vi "DisplayArm.vi"(4 "Init?":bool, 6 "ClosePt":dbl[](array[numeric]), 7 "Field Force":dbl[](array[numeric]), 8 "AnkleTraj":dbl[][](array[numeric]), 9 "CablePos":cluster{"PointInGCS":dbl[][]}[](array[cluster]), 10 "Joint Coord in GCS":dbl[][](array[numeric]), 11 "3D graph in":refnum<k7>) -> (3 "3D graph out":refnum<k7>)   [LabVIEW 2014]
uses:
  <vilib>/Platform/NI_3dgraph.lvlib
  <vilib>/ptbypt/NI_PtbyPt.lvlib
panel:
  in  "sample length":i32=100
  out "LastPlotNum":i32=1
  out "error out":errorcluster
  in  "error in (no error)":errorcluster
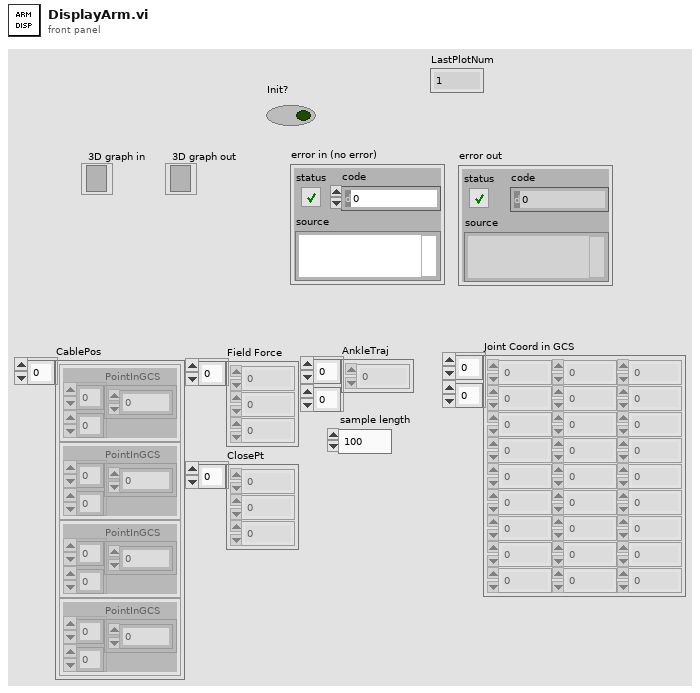
[diagram p1: front panel]
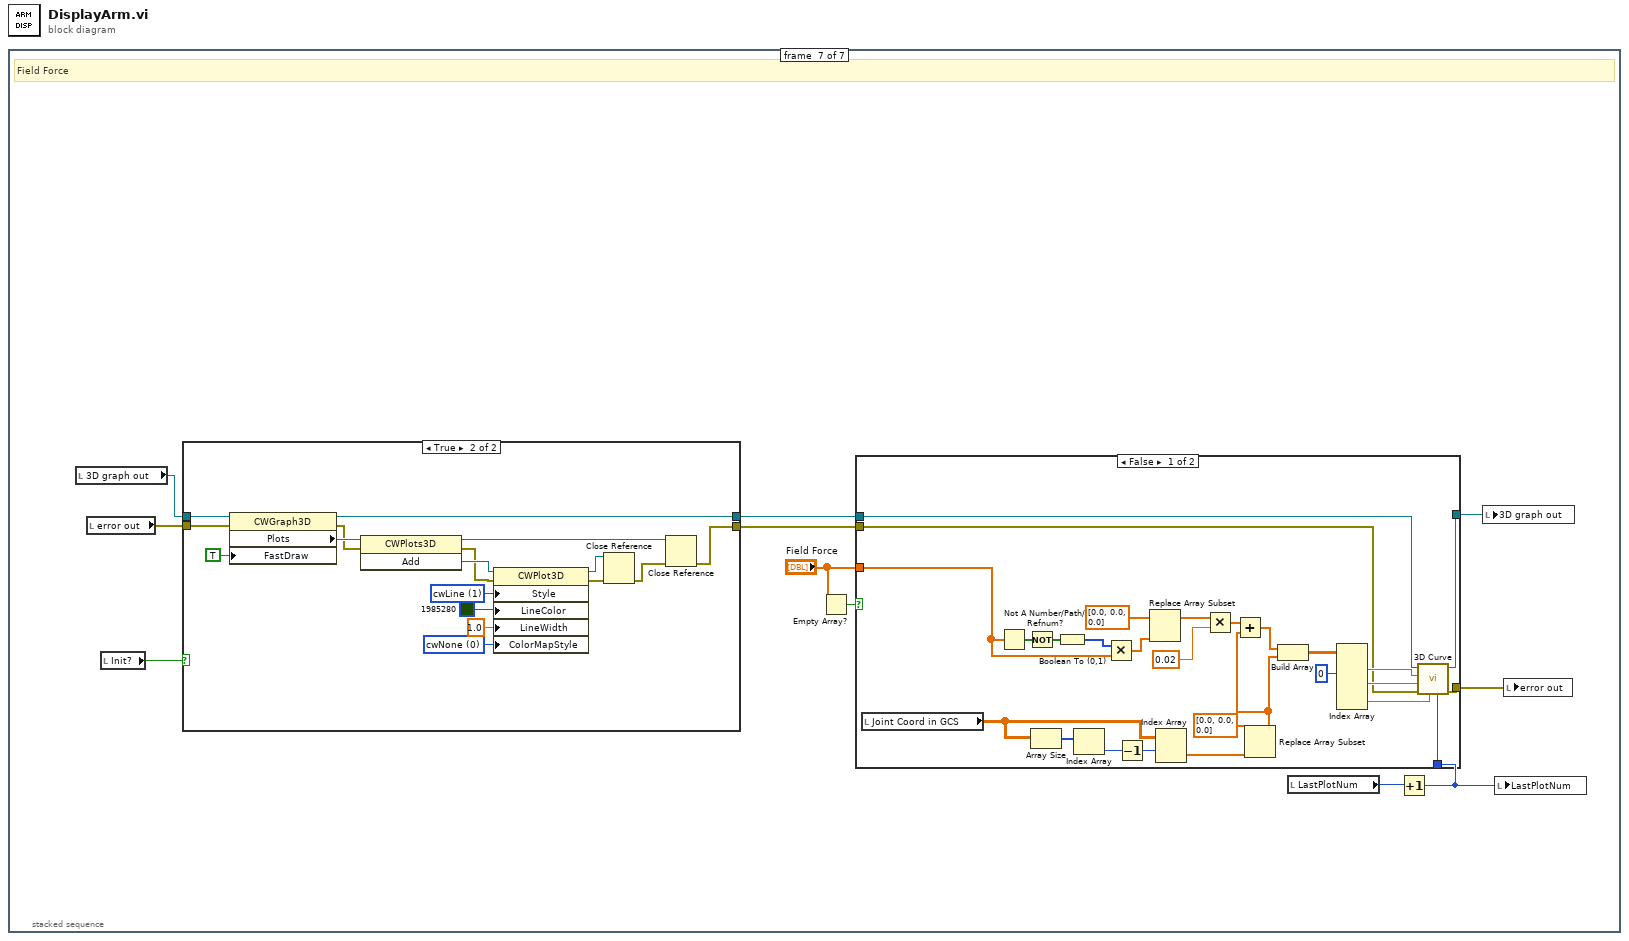
[diagram p0: block diagram]
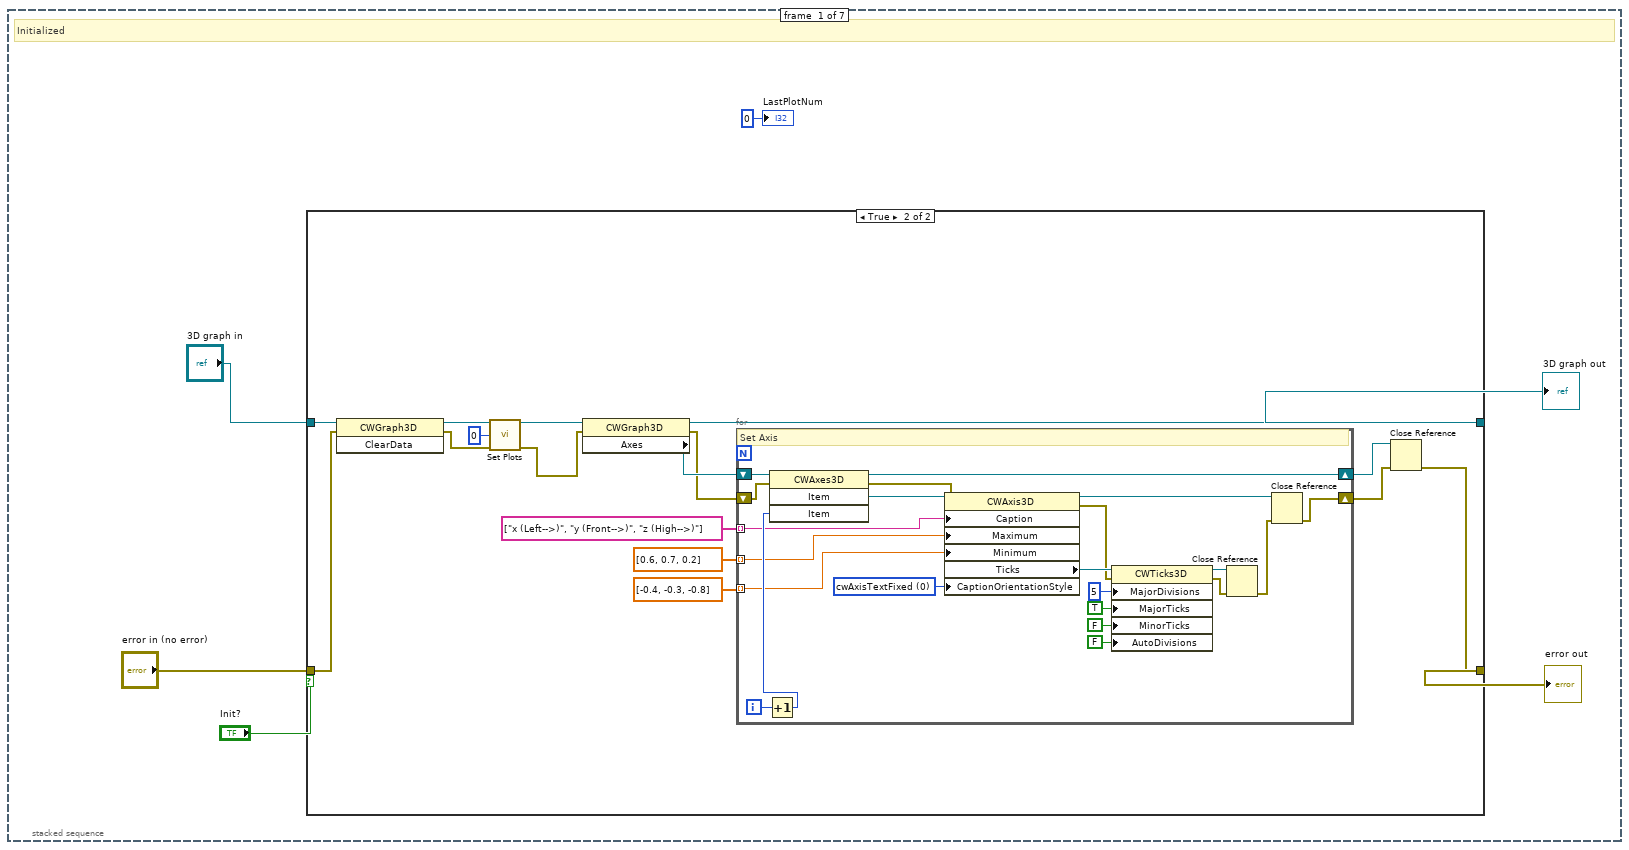
[diagram p2: hidden frame]
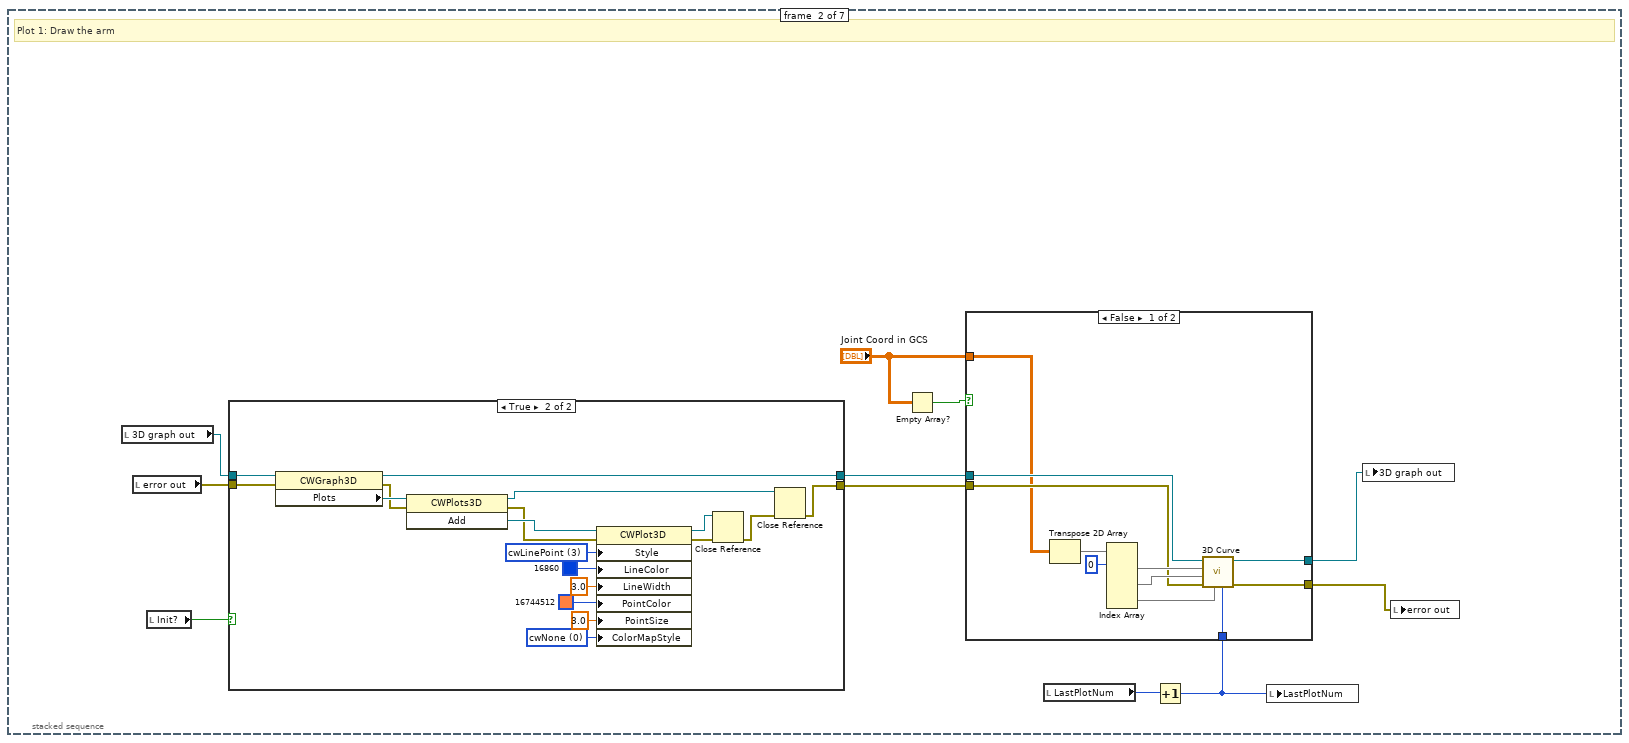
[diagram p4: hidden frame]
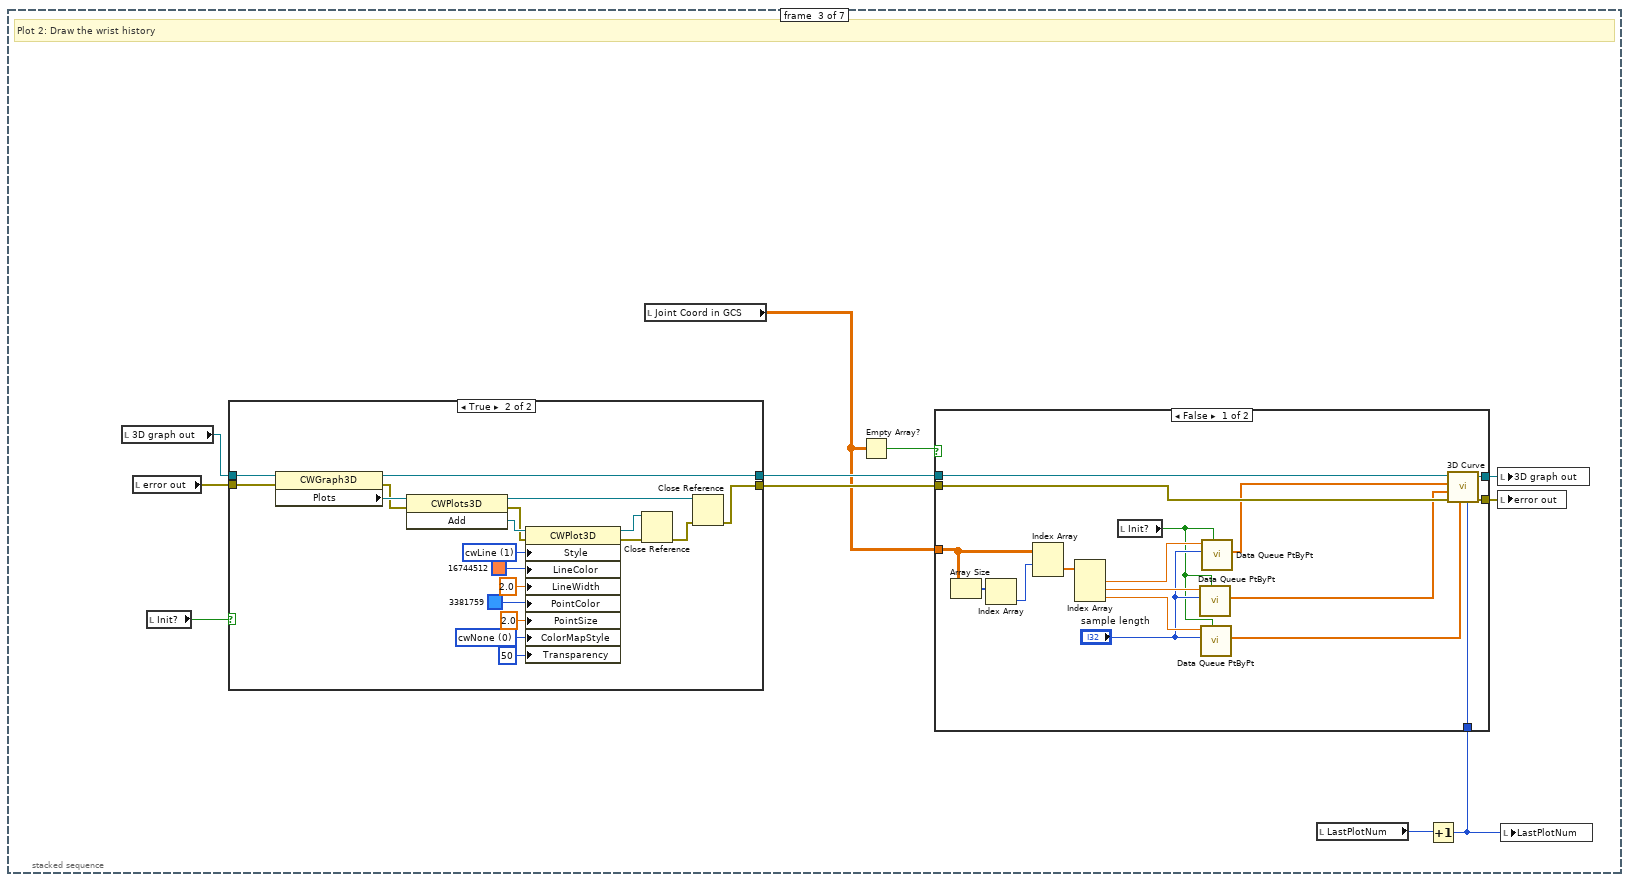
[diagram p7: hidden frame]
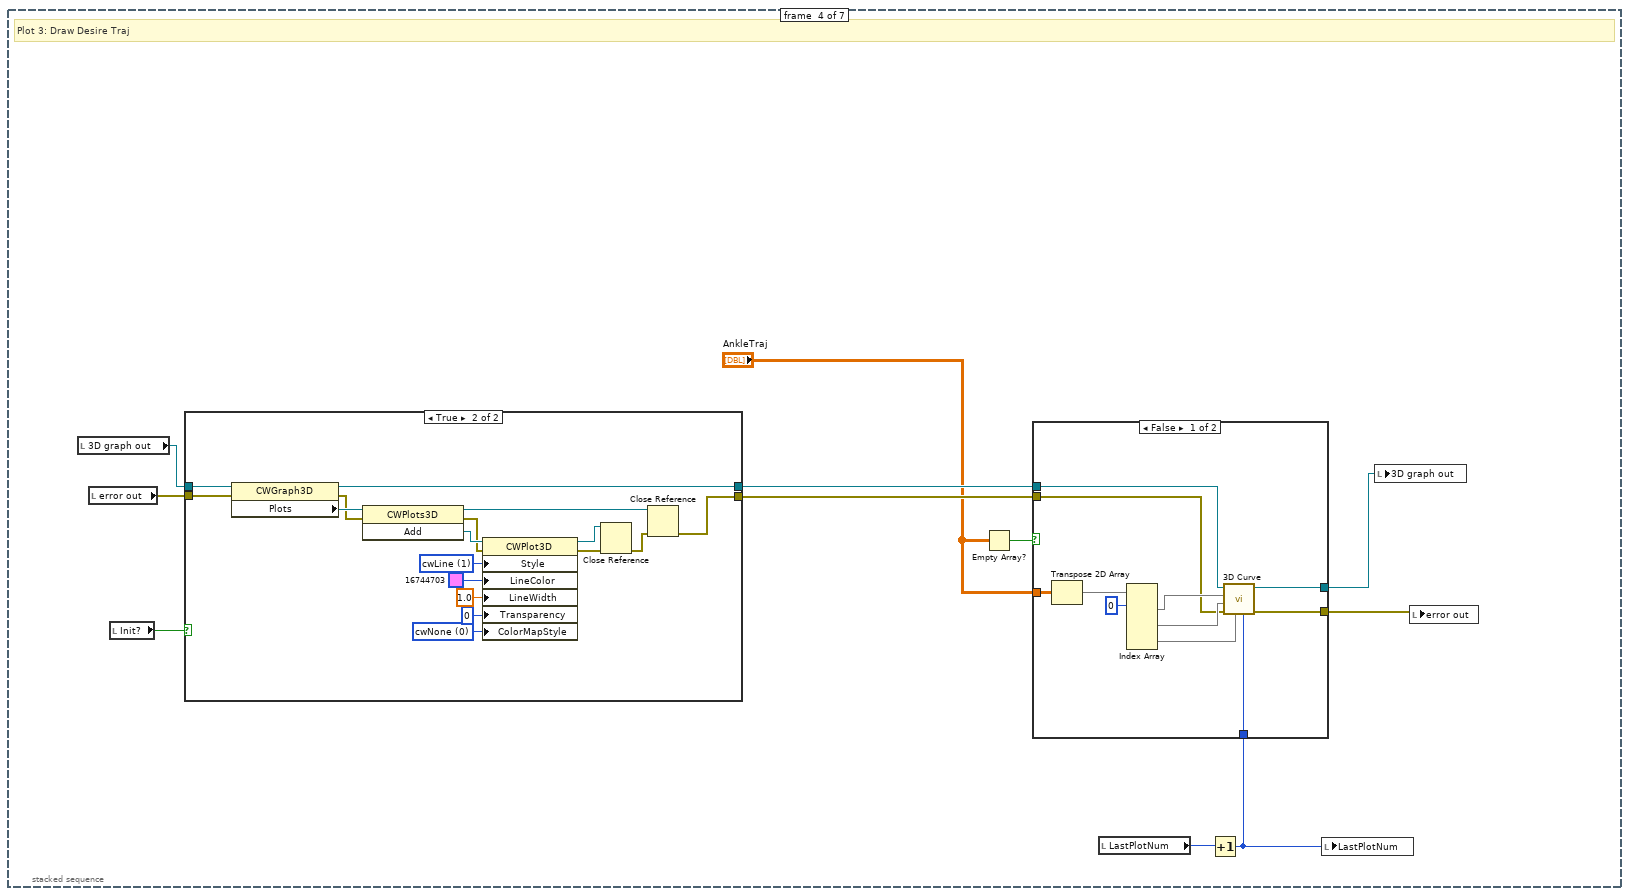
[diagram p10: hidden frame]
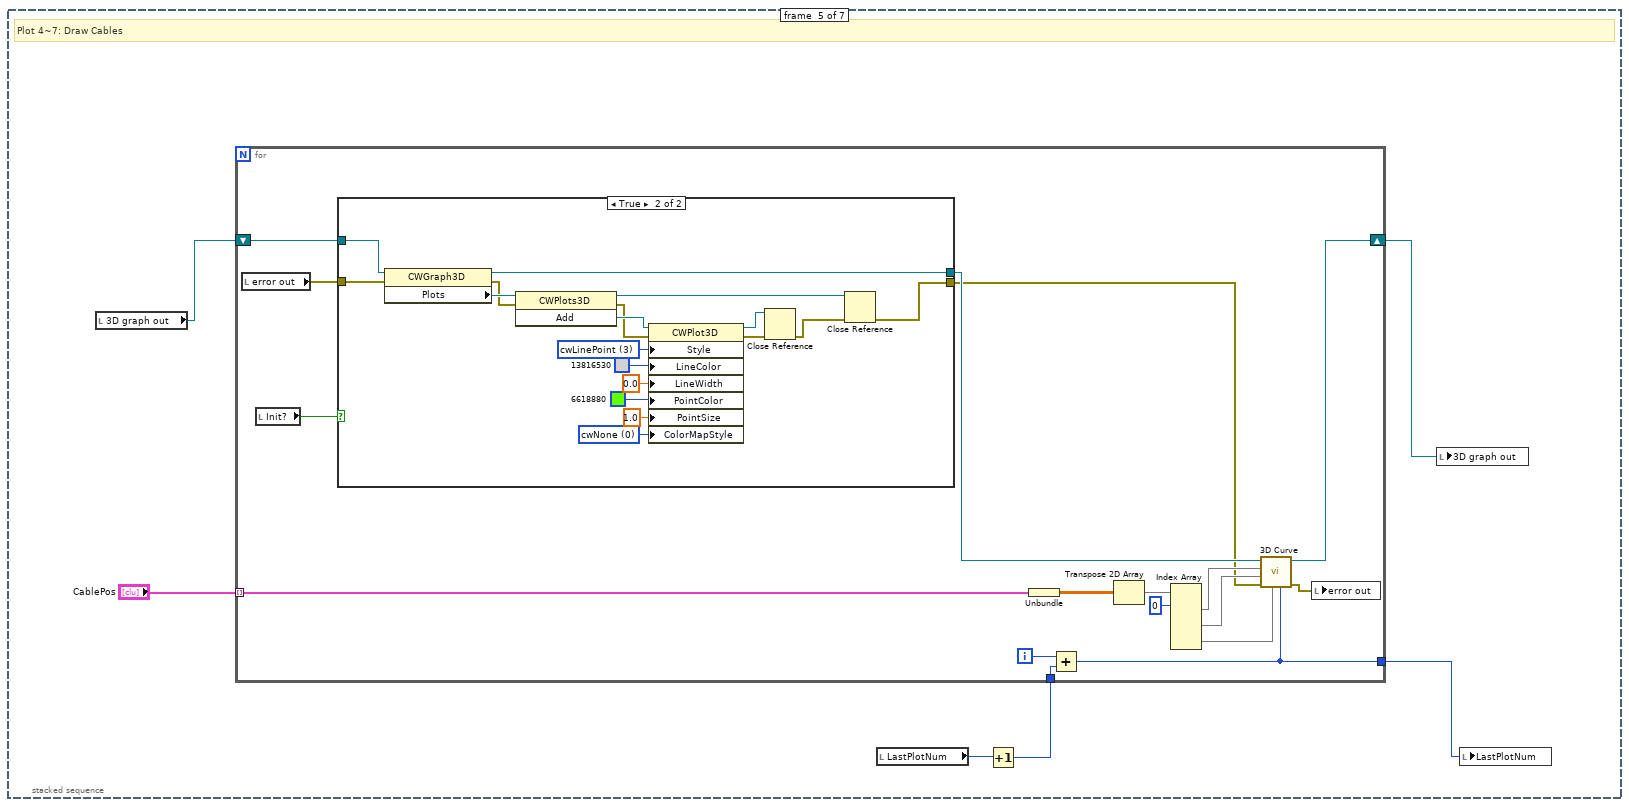
[diagram p13: hidden frame]
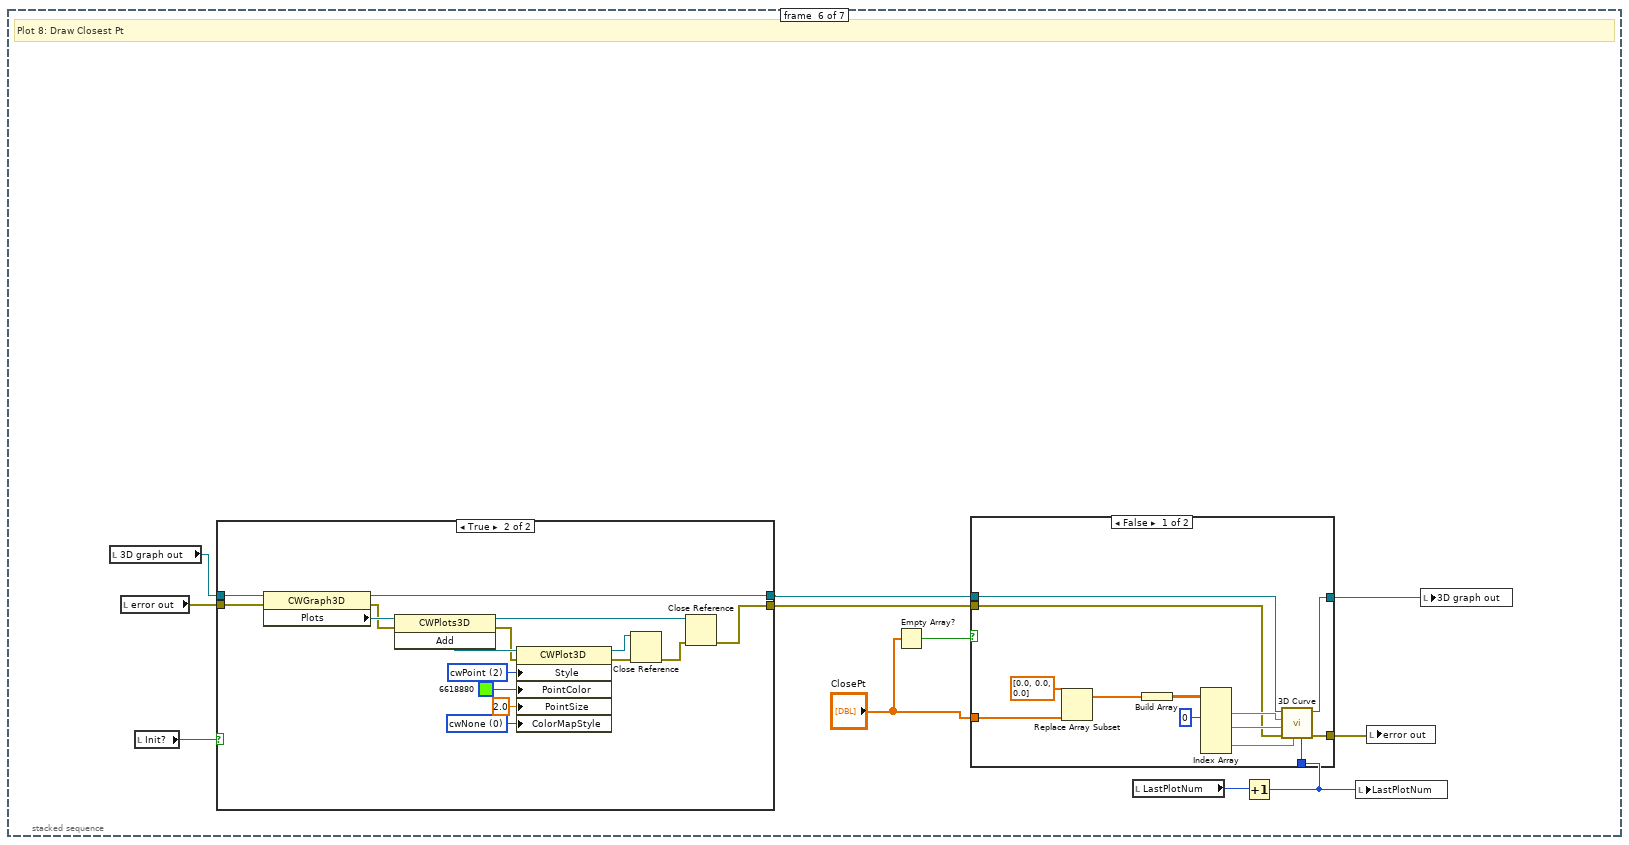
[diagram p15: hidden frame]
diagram:
  n1 = stacked-sequence {
    frame #0 {
      # "Initialized"
      n2 = case shown="True" "Init?" {
        tunnel: "3D graph in" -> [w8 w21]
        tunnel: [w8 w17] -> w5
        tunnel: [w7 w12] -> w3
        tunnel: "error in (no error)" -> [w7 w19]
        frame False {
        }
        frame True {
          n3 = invoke class="CWGraph3D" method="ClearData"(reference=w21, error in=w19) -> (reference out=w20:refnum<k7>, error out=w18:errorcluster)  [unwired: 1 in, 1 out]
          n4 = call <vilib>:"Set Plots.vi"("3D graph"=w20, "# of plots(1)"=0, "error in (no error)"=w18) -> ("3D graph out"=w22:refnum<k7>, "error out"=w13:errorcluster)  [unwired: 11 in]
          n5 = property class="CWGraph3D"(reference=w22, error in=w13) -> (reference out=w17:refnum<k7>, error out=w14:errorcluster, "Axes"=w23:refnum<k7>)
          n6 = for {
            shift-right: [w33] -> w15
            shift-left: w23 -> [w46]
            shift-right: [w34] -> w16
            shift-left: w14 -> [w31]
            tunnel: string[] ["x (Left-->)", "y (Front-->)", "z (High-->)"] -> [w27] mode=indexing
            tunnel: dbl[] [0.6, 0.7, 0.2] -> [w26] mode=indexing
            tunnel: dbl[] [-0.4, -0.3, -0.8] -> [w25] mode=indexing
            i -> [w29]
            w30 = 0 items=["cwAxisTextFixed", "cwAxisTextFaceCamera"] ("CaptionOrientationStyle")
            # "Set Axis"
            n7 = Increment(x=w29) -> (x+1=w28:i32)
            n8 = invoke class="CWAxes3D" method="Item"(reference=w46, error in=w31, "Item"=w28) -> (reference out=w33:refnum<k7>, error out=w32:errorcluster, "Item"=w45:refnum<k7>)  [unwired: 1 in, 1 out]
            n9 = property class="CWAxis3D"(reference=w45, error in=w32, "Caption"=w27, "Maximum"=w26, "Minimum"=w25, "CaptionOrientationStyle"=w30) -> (reference out=w35:refnum<k7>, error out=w38:errorcluster, "Ticks"=w44:refnum<k7>)
            n10 = property class="CWTicks3D"(reference=w44, error in=w38, "MajorDivisions"=5, "MajorTicks"=TRUE, "MinorTicks"=FALSE, "AutoDivisions"=FALSE) -> (reference out=w37:refnum<k7>, error out=w39:errorcluster)
            n11 = Close Reference(reference=w37, error in (no error)=w39) -> (error out=w36:errorcluster)
            n12 = Close Reference(reference=w35, error in (no error)=w36) -> (error out=w34:errorcluster)
          }
          n13 = Close Reference(reference=w15, error in (no error)=w16) -> (error out=w12:errorcluster)
        }
      }
      "3D graph out" <- w5
      "error out" <- w3
      "LastPlotNum" <- 0 ("LastPlotNum 2")
    }
    frame #1 {
      # "Plot 1: Draw the arm"
      n14 = local read "3D graph out"() -> (w55:refnum<k7>)
      n15 = local read "error out"() -> (w56:errorcluster)
      n16 = local read "Init?"() -> (w49:bool)
      n17 = case shown="True" w49 {
        tunnel: w56 -> [w71 w84]
        tunnel: w55 -> [w72 w79]
        tunnel: [w72 w78] -> w54
        tunnel: [w71 w73] -> w53
        frame False {
        }
        frame True {
          w77 = 0 items=["cwNone", "cwShaded", "cwColorSpectrum", "cwGrayScale", "cwCustom"] ("ColorMapStyle")
          w90 = 3 items=["cwLine"=1, "cwPoint"=2, "cwLinePoint"=3, "cwHiddenLine"=4, "cwSurface"=5, "cwSurfaceLine"=6, "cwSurfaceNormal"=7, "cwContourLine"=8, "cwSurfaceContour"=9] ("Style")
          n18 = property class="CWGraph3D"(reference=w79, error in=w84) -> (reference out=w78:refnum<k7>, error out=w87:errorcluster, "Plots"=w88:refnum<k7>)
          n19 = invoke class="CWPlots3D" method="Add"(reference=w88, error in=w87) -> (reference out=w75:refnum<k7>, error out=w76:errorcluster, "Add"=w89:refnum<k7>)  [unwired: 1 in]
          n20 = property class="CWPlot3D"(reference=w89, error in=w76, "Style"=w90, "LineColor"=u32 16860, "LineWidth"=3.0, "PointColor"=u32 16744512, "PointSize"=3.0 ("LineWidth"), "ColorMapStyle"=w77) -> (reference out=w85:refnum<k7>, error out=w86:errorcluster)
          n21 = Close Reference(reference=w85, error in (no error)=w86) -> (error out=w74:errorcluster)
          n22 = Close Reference(reference=w75, error in (no error)=w74) -> (error out=w73:errorcluster)
        }
      }
      n23 = Empty Array?(array="Joint Coord in GCS") -> (empty?=w47:bool)
      n24 = local read "LastPlotNum"() -> (w51:i32)
      n25 = Increment(x=w51) -> (x+1=w50:i32)
      n26 = case shown="False" w47 {
        tunnel: [w63 w70] -> w57
        tunnel: w54 -> [w62 w70]
        tunnel: w53 -> [w61 w69]
        tunnel: [w60 w69] -> w52
        tunnel: w50 -> [w59 _]
        tunnel: "Joint Coord in GCS" -> [w58 _]
        frame False {
          n27 = Transpose 2D Array(2D array=w58) -> (transposed array=w64:dbl[][])
          n28 = Index Array(array=w64, index (row) #1=0 ("index (row)")) -> (element #1=w66:dbl[], element #2=w67:dbl[], element #3=w68:dbl[])  [unwired: 5 in]
          n29 = call <vilib>:"3D Curve.vi"("plot number (1)"=w59, "z vector"=w68, "error in (no error)"=w61, "y vector"=w67, "x vector"=w66, "3D graph"=w62) -> ("error out"=w60:errorcluster, "3D graph out"=w63:refnum<k7>)  [unwired: 4 in]
        }
        frame True {
        }
      }
      n30 = local write "LastPlotNum"(w50) -> ()
      n31 = local write "3D graph out"(w57) -> ()
      n32 = local write "error out"(w52) -> ()
    }
    frame #2 {
      # "Plot 2: Draw the wrist history"
      n33 = local read "3D graph out"() -> (w99:refnum<k7>)
      n34 = local read "error out"() -> (w100:errorcluster)
      n35 = local read "Init?"() -> (w94:bool)
      n36 = case shown="True" w94 {
        tunnel: w100 -> [w121 w134]
        tunnel: w99 -> [w122 w129]
        tunnel: [w122 w128] -> w98
        tunnel: [w121 w123] -> w97
        frame False {
        }
        frame True {
          w127 = 0 items=["cwNone", "cwShaded", "cwColorSpectrum", "cwGrayScale", "cwCustom"] ("ColorMapStyle")
          w141 = 1 items=["cwLine"=1, "cwPoint"=2, "cwLinePoint"=3, "cwHiddenLine"=4, "cwSurface"=5, "cwSurfaceLine"=6, "cwSurfaceNormal"=7, "cwContourLine"=8, "cwSurfaceContour"=9] ("Style")
          n37 = property class="CWGraph3D"(reference=w129, error in=w134) -> (reference out=w128:refnum<k7>, error out=w138:errorcluster, "Plots"=w139:refnum<k7>)
          n38 = invoke class="CWPlots3D" method="Add"(reference=w139, error in=w138) -> (reference out=w137:refnum<k7>, error out=w125:errorcluster, "Add"=w140:refnum<k7>)  [unwired: 1 in]
          n39 = property class="CWPlot3D"(reference=w140, error in=w125, "Style"=w141, "LineColor"=u32 16744512, "LineWidth"=2.0, "PointColor"=u32 3381759, "PointSize"=2.0 ("LineWidth"), "ColorMapStyle"=w127, "Transparency"=50) -> (reference out=w135:refnum<k7>, error out=w136:errorcluster)
          n40 = Close Reference(reference=w135, error in (no error)=w136) -> (error out=w124:errorcluster)
          n41 = Close Reference(reference=w137, error in (no error)=w124) -> (error out=w123:errorcluster)
        }
      }
      n42 = local read "Joint Coord in GCS"() -> (w92:dbl[][])
      n43 = Empty Array?(array=w92) -> (empty?=w91:bool)
      n44 = local read "LastPlotNum"() -> (w93:i32)
      n45 = Increment(x=w93) -> (x+1=w95:i32)
      n46 = case shown="False" w91 {
        tunnel: [w118 w120] -> w101
        tunnel: w98 -> [w117 w120]
        tunnel: w97 -> [w116 w119]
        tunnel: [w115 w119] -> w96
        tunnel: w95 -> [w114 _]
        tunnel: w92 -> [w113 _]
        frame False {
          n47 = Array Size(array=w113) -> (size(s)=w112:i32[])
          n48 = Index Array(array=w112) -> (element=w111:i32)  [unwired: 1 in]
          n49 = Index Array(array=w113, index (row)=w111) -> (element=w110:dbl[])  [unwired: 1 in]
          n50 = Index Array(array=w110) -> (element #1=w107:dbl, element #2=w108:dbl, element #3=w109:dbl)  [unwired: 3 in]
          n51 = local read "Init?"() -> (w102:bool)
          n52 = call <vilib>:"Data Queue PtByPt.vi"("initialize"=w102, "sample length"="sample length", "input data point"=w108) -> ("Current Queue"=w104:dbl[])  [unwired: 4 in, 4 out]
          n53 = call <vilib>:"Data Queue PtByPt.vi"("initialize"=w102, "sample length"="sample length", "input data point"=w109) -> ("Current Queue"=w103:dbl[])  [unwired: 4 in, 4 out]
          n54 = call <vilib>:"Data Queue PtByPt.vi"("initialize"=w102, "sample length"="sample length", "input data point"=w107) -> ("Current Queue"=w105:dbl[])  [unwired: 4 in, 4 out]
          n55 = call <vilib>:"3D Curve.vi"("plot number (1)"=w114, "z vector"=w103, "error in (no error)"=w116, "y vector"=w104, "x vector"=w105, "3D graph"=w117) -> ("error out"=w115:errorcluster, "3D graph out"=w118:refnum<k7>)  [unwired: 4 in]
        }
        frame True {
        }
      }
      n56 = local write "3D graph out"(w101) -> ()
      n57 = local write "error out"(w96) -> ()
      n58 = local write "LastPlotNum"(w95) -> ()
    }
    frame #3 {
      # "Plot 3: Draw Desire Traj"
      n59 = local read "3D graph out"() -> (w150:refnum<k7>)
      n60 = local read "error out"() -> (w151:errorcluster)
      n61 = local read "Init?"() -> (w146:bool)
      n62 = case shown="True" w146 {
        tunnel: w151 -> [w166 w177]
        tunnel: w150 -> [w167 w174]
        tunnel: [w167 w173] -> w149
        tunnel: [w166 w168] -> w145
        frame False {
        }
        frame True {
          w171 = 0 items=["cwNone", "cwShaded", "cwColorSpectrum", "cwGrayScale", "cwCustom"] ("ColorMapStyle")
          w184 = 1 items=["cwLine"=1, "cwPoint"=2, "cwLinePoint"=3, "cwHiddenLine"=4, "cwSurface"=5, "cwSurfaceLine"=6, "cwSurfaceNormal"=7, "cwContourLine"=8, "cwSurfaceContour"=9] ("Style")
          n63 = property class="CWGraph3D"(reference=w174, error in=w177) -> (reference out=w173:refnum<k7>, error out=w181:errorcluster, "Plots"=w182:refnum<k7>)
          n64 = invoke class="CWPlots3D" method="Add"(reference=w182, error in=w181) -> (reference out=w180:refnum<k7>, error out=w170:errorcluster, "Add"=w183:refnum<k7>)  [unwired: 1 in]
          n65 = property class="CWPlot3D"(reference=w183, error in=w170, "Style"=w184, "LineColor"=u32 16744703, "LineWidth"=1.0, "Transparency"=0, "ColorMapStyle"=w171) -> (reference out=w178:refnum<k7>, error out=w179:errorcluster)
          n66 = Close Reference(reference=w178, error in (no error)=w179) -> (error out=w169:errorcluster)
          n67 = Close Reference(reference=w180, error in (no error)=w169) -> (error out=w168:errorcluster)
        }
      }
      n68 = Empty Array?(array="AnkleTraj") -> (empty?=w143:bool)
      n69 = local read "LastPlotNum"() -> (w148:i32)
      n70 = Increment(x=w148) -> (x+1=w147:i32)
      n71 = case shown="False" w143 {
        tunnel: "AnkleTraj" -> [w163 _]
        tunnel: [w157 w165] -> w152
        tunnel: w149 -> [w156 w165]
        tunnel: w147 -> [w155 _]
        tunnel: w145 -> [w154 w164]
        tunnel: [w153 w164] -> w144
        frame False {
          n72 = Transpose 2D Array(2D array=w163) -> (transposed array=w158:dbl[][])
          n73 = Index Array(array=w158, index (row) #1=0 ("index (row)")) -> (element #1=w160:dbl[], element #2=w161:dbl[], element #3=w162:dbl[])  [unwired: 5 in]
          n74 = call <vilib>:"3D Curve.vi"("plot number (1)"=w155, "z vector"=w162, "error in (no error)"=w154, "y vector"=w161, "x vector"=w160, "3D graph"=w156) -> ("error out"=w153:errorcluster, "3D graph out"=w157:refnum<k7>)  [unwired: 4 in]
        }
        frame True {
        }
      }
      n75 = local write "LastPlotNum"(w147) -> ()
      n76 = local write "3D graph out"(w152) -> ()
      n77 = local write "error out"(w144) -> ()
    }
    frame #4 {
      # "Plot 4~7: Draw Cables"
      n78 = local read "3D graph out"() -> (w187:refnum<k7>)
      n79 = local read "LastPlotNum"() -> (w188:i32)
      n80 = Increment(x=w188) -> (x+1=w186:i32)
      n81 = for {
        tunnel: "CablePos" -> [w205] mode=indexing
        shift-right: [w203] -> w189
        shift-left: w187 -> [w196]
        tunnel: w186 -> [w194]
        tunnel: [w193] -> w185
        i -> [w199]
        n82 = local read "error out"() -> (w198:errorcluster)
        n83 = local read "Init?"() -> (w197:bool)
        n84 = case shown="True" w197 {
          tunnel: w198 -> [w209 w220]
          tunnel: [w208 w215] -> w195
          tunnel: [w209 w210] -> w192
          tunnel: w196 -> [w208 w213]
          frame False {
          }
          frame True {
            w214 = 0 items=["cwNone", "cwShaded", "cwColorSpectrum", "cwGrayScale", "cwCustom"] ("ColorMapStyle")
            w227 = 3 items=["cwLine"=1, "cwPoint"=2, "cwLinePoint"=3, "cwHiddenLine"=4, "cwSurface"=5, "cwSurfaceLine"=6, "cwSurfaceNormal"=7, "cwContourLine"=8, "cwSurfaceContour"=9] ("Style")
            n85 = property class="CWGraph3D"(reference=w213, error in=w220) -> (reference out=w215:refnum<k7>, error out=w224:errorcluster, "Plots"=w225:refnum<k7>)
            n86 = invoke class="CWPlots3D" method="Add"(reference=w225, error in=w224) -> (reference out=w223:refnum<k7>, error out=w212:errorcluster, "Add"=w226:refnum<k7>)  [unwired: 1 in]
            n87 = property class="CWPlot3D"(reference=w226, error in=w212, "Style"=w227, "LineColor"=u32 13816530, "LineWidth"=0.0, "PointColor"=u32 6618880, "PointSize"=1.0 ("LineWidth"), "ColorMapStyle"=w214) -> (reference out=w221:refnum<k7>, error out=w222:errorcluster)
            n88 = Close Reference(reference=w221, error in (no error)=w222) -> (error out=w211:errorcluster)
            n89 = Close Reference(reference=w223, error in (no error)=w211) -> (error out=w210:errorcluster)
          }
        }
        n90 = Unbundle(w205) -> ("PointInGCS"=w204:dbl[][])
        n91 = Add(x=w199, y=w194) -> (x+y=w193:i32)
        n92 = Transpose 2D Array(2D array=w204) -> (transposed array=w206:dbl[][])
        n93 = Index Array(array=w206, index (row) #1=0 ("index (row)")) -> (element #1=w202:dbl[], element #2=w201:dbl[], element #3=w200:dbl[])  [unwired: 5 in]
        n94 = call <vilib>:"3D Curve.vi"("plot number (1)"=w193, "z vector"=w200, "error in (no error)"=w192, "y vector"=w201, "x vector"=w202, "3D graph"=w195) -> ("error out"=w191:errorcluster, "3D graph out"=w203:refnum<k7>)  [unwired: 4 in]
        n95 = local write "error out"(w191) -> ()
      }
      n96 = local write "3D graph out"(w189) -> ()
      n97 = local write "LastPlotNum"(w185) -> ()
    }
    frame #5 {
      # "Plot 8: Draw Closest Pt"
      n98 = local read "3D graph out"() -> (w236:refnum<k7>)
      n99 = local read "error out"() -> (w237:errorcluster)
      n100 = local read "Init?"() -> (w235:bool)
      n101 = case shown="True" w235 {
        tunnel: w237 -> [w254 w264]
        tunnel: w236 -> [w255 w261]
        tunnel: [w255 w260] -> w234
        tunnel: [w254 w256] -> w231
        frame False {
        }
        frame True {
          w259 = 0 items=["cwNone", "cwShaded", "cwColorSpectrum", "cwGrayScale", "cwCustom"] ("ColorMapStyle")
          w271 = 2 items=["cwLine"=1, "cwPoint"=2, "cwLinePoint"=3, "cwHiddenLine"=4, "cwSurface"=5, "cwSurfaceLine"=6, "cwSurfaceNormal"=7, "cwContourLine"=8, "cwSurfaceContour"=9] ("Style")
          n102 = property class="CWGraph3D"(reference=w261, error in=w264) -> (reference out=w260:refnum<k7>, error out=w268:errorcluster, "Plots"=w269:refnum<k7>)
          n103 = invoke class="CWPlots3D" method="Add"(reference=w269, error in=w268) -> (reference out=w267:refnum<k7>, error out=w258:errorcluster, "Add"=w270:refnum<k7>)  [unwired: 1 in]
          n104 = property class="CWPlot3D"(reference=w270, error in=w258, "Style"=w271, "PointColor"=u32 6618880, "PointSize"=2.0 ("LineWidth"), "ColorMapStyle"=w259) -> (reference out=w265:refnum<k7>, error out=w266:errorcluster)
          n105 = Close Reference(reference=w265, error in (no error)=w266) -> (error out=w257:errorcluster)
          n106 = Close Reference(reference=w267, error in (no error)=w257) -> (error out=w256:errorcluster)
        }
      }
      n107 = Empty Array?(array="ClosePt") -> (empty?=w228:bool)
      n108 = local read "LastPlotNum"() -> (w233:i32)
      n109 = Increment(x=w233) -> (x+1=w232:i32)
      n110 = case shown="False" w228 {
        tunnel: "ClosePt" -> [w250 _]
        tunnel: [w243 w253] -> w238
        tunnel: w234 -> [w242 w253]
        tunnel: w232 -> [w241 _]
        tunnel: w231 -> [w240 w252]
        tunnel: [w239 w252] -> w230
        frame False {
          n111 = Replace Array Subset(array=dbl[] [0.0, 0.0, 0.0], new element=w250) -> (w249:dbl[])  [unwired: 1 in]
          n112 = Build Array(w249) -> (w248:dbl[][])
          n113 = Index Array(array=w248, index (col) #1=0 ("disabled index (col)")) -> (element #1=w246:dbl[], element #2=w245:dbl[], element #3=w244:dbl[])  [unwired: 5 in]
          n114 = call <vilib>:"3D Curve.vi"("plot number (1)"=w241, "z vector"=w244, "error in (no error)"=w240, "y vector"=w245, "x vector"=w246, "3D graph"=w242) -> ("error out"=w239:errorcluster, "3D graph out"=w243:refnum<k7>)  [unwired: 4 in]
        }
        frame True {
        }
      }
      n115 = local write "LastPlotNum"(w232) -> ()
      n116 = local write "error out"(w230) -> ()
      n117 = local write "3D graph out"(w238) -> ()
    }
    frame #6 {
      # "Field Force"
      n118 = local read "3D graph out"() -> (w280:refnum<k7>)
      n119 = local read "error out"() -> (w281:errorcluster)
      n120 = local read "Init?"() -> (w279:bool)
      n121 = case shown="True" w279 {
        tunnel: w281 -> [w312 w323]
        tunnel: w280 -> [w313 w320]
        tunnel: [w313 w319] -> w278
        tunnel: [w312 w314] -> w275
        frame False {
        }
        frame True {
          w318 = 0 items=["cwNone", "cwShaded", "cwColorSpectrum", "cwGrayScale", "cwCustom"] ("ColorMapStyle")
          w330 = 1 items=["cwLine"=1, "cwPoint"=2, "cwLinePoint"=3, "cwHiddenLine"=4, "cwSurface"=5, "cwSurfaceLine"=6, "cwSurfaceNormal"=7, "cwContourLine"=8, "cwSurfaceContour"=9] ("Style")
          n122 = property class="CWGraph3D"(reference=w320, error in=w323, "FastDraw"=TRUE) -> (reference out=w319:refnum<k7>, error out=w327:errorcluster, "Plots"=w328:refnum<k7>)
          n123 = invoke class="CWPlots3D" method="Add"(reference=w328, error in=w327) -> (reference out=w326:refnum<k7>, error out=w316:errorcluster, "Add"=w329:refnum<k7>)  [unwired: 1 in]
          n124 = property class="CWPlot3D"(reference=w329, error in=w316, "Style"=w330, "LineColor"=u32 1985280, "LineWidth"=1.0, "ColorMapStyle"=w318) -> (reference out=w324:refnum<k7>, error out=w325:errorcluster)
          n125 = Close Reference(reference=w324, error in (no error)=w325) -> (error out=w315:errorcluster)
          n126 = Close Reference(reference=w326, error in (no error)=w315) -> (error out=w314:errorcluster)
        }
      }
      n127 = Empty Array?(array="Field Force") -> (empty?=w272:bool)
      n128 = local read "LastPlotNum"() -> (w277:i32)
      n129 = Increment(x=w277) -> (x+1=w276:i32)
      n130 = case shown="False" w272 {
        tunnel: [w288 w311] -> w282
        tunnel: w278 -> [w287 w311]
        tunnel: w276 -> [w286 _]
        tunnel: w275 -> [w285 w310]
        tunnel: [w284 w310] -> w274
        tunnel: "Field Force" -> [w283 _]
        frame False {
          n131 = local read "Joint Coord in GCS"() -> (w309:dbl[][])
          n132 = Not A Number/Path/Refnum?(number/path/refnum=w283) -> (NaN/Path/Refnum?=w292:bool[])
          n133 = Not(x=w292) -> (.not. x?=w291:bool[])
          n134 = Array Size(array=w309) -> (size(s)=w298:i32[])
          n135 = Boolean To (0,1)(Boolean=w291) -> (0, 1=w290:i16[])
          n136 = Index Array(array=w298) -> (element=w300:i32)  [unwired: 1 in]
          n137 = Multiply(x=w290, y=w283) -> (x*y=w289:dbl[])
          n138 = Decrement(x=w300) -> (x-1=w299:i32)
          n139 = Replace Array Subset(array=dbl[] [0.0, 0.0, 0.0], new element=w289) -> (w305:dbl[])  [unwired: 1 in]
          n140 = Index Array(array=w309, index (row)=w299) -> (element=w307:dbl[])  [unwired: 1 in]
          n141 = Multiply(x=w305, y=0.02) -> (x*y=w297:dbl[])
          n142 = Replace Array Subset(array=dbl[] [0.0, 0.0, 0.0], new element=w307) -> (w308:dbl[])  [unwired: 1 in]
          n143 = Add(x=w297, y=w308) -> (x+y=w294:dbl[])
          n144 = Build Array(w294, w308) -> (w295:dbl[][])
          n145 = Index Array(array=w295, index (col) #1=0 ("disabled index (col)")) -> (element #1=w301:dbl[], element #2=w302:dbl[], element #3=w303:dbl[])  [unwired: 5 in]
          n146 = call <vilib>:"3D Curve.vi"("plot number (1)"=w286, "z vector"=w303, "error in (no error)"=w285, "y vector"=w302, "x vector"=w301, "3D graph"=w287) -> ("error out"=w284:errorcluster, "3D graph out"=w288:refnum<k7>)  [unwired: 4 in]
        }
        frame True {
        }
      }
      n147 = local write "3D graph out"(w282) -> ()
      n148 = local write "LastPlotNum"(w276) -> ()
      n149 = local write "error out"(w274) -> ()
    }
  }
